vi "LabConcentrationGraph.vi"(1 "L*a*b*":dbl[][](array[numeric])) -> (0 "L*a*b Variation":T1)   [LabVIEW 2013]
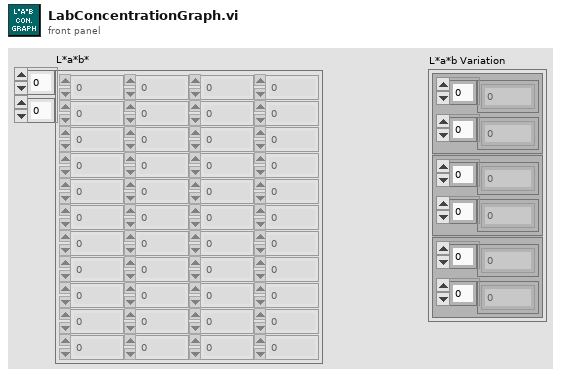
[diagram p1: front panel]
types:
  T1 = cluster{cluster{i32[], dbl[]}, cluster{i32[], dbl[]}, cluster{i32[], dbl[]}}
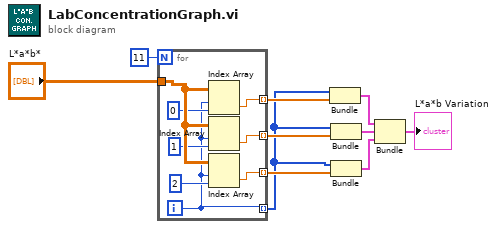
[diagram p0: block diagram]
diagram:
  n1 = for {
    N: 11 -> [_]
    tunnel: "L*a*b*" -> [w18]
    tunnel: [w17] -> w5 mode=indexing
    tunnel: [w16] -> w4 mode=indexing
    tunnel: [w15] -> w3 mode=indexing
    tunnel: [w11] -> w2 mode=indexing
    i -> [w11]
    n2 = Index Array(array=w18, index (row)=w11, index (col)=0 ("index (row)")) -> (element=w17:dbl)
    n3 = Index Array(array=w18, index (row)=w11, index (col)=1 ("index (row)")) -> (element=w16:dbl)
    n4 = Index Array(array=w18, index (row)=w11, index (col)=2 ("index (row)")) -> (element=w15:dbl)
  }
  n5 = Bundle(w2, w5) -> (w8:cluster{i32[], dbl[]})  [unwired: 1 in]
  n6 = Bundle(w2, w4) -> (w7:cluster{i32[], dbl[]})  [unwired: 1 in]
  n7 = Bundle(w2, w3) -> (w6:cluster{i32[], dbl[]})  [unwired: 1 in]
  n8 = Bundle(w8, w7, w6) -> (→"L*a*b Variation":T1)  [unwired: 1 in]
